vi "NI9239_Producer_Consumer.vi"() -> ()   [LabVIEW 2018]
doc: "Use this template to build a producer/consumer design pattern. Use this template when you need to execute a process, such as data analysis, when a data source, such as a triggered acquisition, produces data at an uneven rate and you need to execute the process when the data becomes available."
uses:
  <vilib>/DAQmx/read.llb/DAQmx Read (Analog 1D Wfm NChan NSamp).vi
  <vilib>/Utility/file.llb/Write Delimited Spreadsheet (string).vi
  <vilib>/DAQmx/miscellaneous.llb/DAQmx Fill In Error Info.vi
  <vilib>/ptbypt/NI_PtbyPt.lvlib
panel:
  out "Directemp (C)":string
  in  "max voltage value":dbl=1.0 format="%0.2f"
  in  "min voltage value":dbl=-1.0 format="%0.2f"
  out "Tot. samples/sec":dbl=1397.9644232175574 format="%_5g"
  out "Array Size":dbl=1000.0
  out "Data Points/Sec":dbl=1.3979644232175574 format="%#_4g"
  in  "samples \nper channel":i32=1000
  in  "samp./ch.":i32=1000
  out "pH output":dbl=3.8843481913333946
  out "error out":errorcluster
  in  "stop":bool
  out "Total Data Points":i32=1166
  out "data":waveform(dbl)[](array[waveform])=[{"t0"=timestamp(3649432382.4522414 s since 1904-01-01), "dt"=0.00062, "Y"=array[1000 elements], "attributes"=variant("NI_ChannelName"=variant(string "Voltage"), "NI_UnitDescription"=variant(string "Volts"))}]
  out "std dev (mV)":dbl=0.018712825305373 format="%0.4f"
  in  "stdev samples":i32=100
  out "Voltage":dbl[][](array[numeric])=[[-0.1627778496], [-0.162776595675], [-0.16276029465], [-0.162771579975], [-0.162937098075], [-0.163070014125], [-0.16318662915], [-0.163360924725], [-0.16341985920000002], [-0.163636788225], [-0.163847447625], [-0.16384870155], [-0.1640969787], [-0.164038044225], [-0.164186007375], [-0.16422487905], [-0.16418475345], [-0.164040552075], [-0.163872526125], [-0.16373459437500001], [-0.163659358875], [-0.16361797935], [-0.163498856475], [-0.16323177045], [-0.162989762925], [-0.162989762925], [-0.1628932107], [-0.16271515335], [-0.162728946525], [-0.1627728339], [-0.162756532875], [-0.1629533991], [-0.16315402710000002], [-0.1632443097], [-0.163333338375], [-0.16343741415000002], [-0.16373584830000001], [-0.163947761625], [-0.16401421965000001], [-0.1641170415], [-0.1641972927], [-0.16433522445], [-0.164223625125], [-0.1641521514], [-0.164103248325], [-0.16398914115000002], [-0.1638261309], [-0.16371076980000002], [-0.16358286945], [-0.163365940425], [-0.1630988544], [-0.163012333575], [-0.16287816360000001], [-0.16283051445], [-0.162787881], [-0.162787881], [-0.162723930825], [-0.16286186257500002], [-0.163002302175], [-0.1631139015], [-0.163197914475], [-0.16327691175], [-0.16339728855], [-0.163691960925], [-0.163852463325], [-0.163980363675], [-0.164110771875], [-0.164108264025], [-0.16428757530000002], [-0.16424494185], [-0.164168452425], [-0.16408945515], [-0.163952777325], [-0.16377848175], [-0.1636555971], [-0.163461238725], [-0.163373463975], [-0.1631740899], [-0.16308631515], [-0.162934590225], [-0.16287690967500001], [-0.162746501475], [-0.162676281675], [-0.162733962225], [-0.162756532875], [-0.1630186032], [-0.16309133085], [-0.16329697455], [-0.1633596708], [-0.1635101418], [-0.16373208652500001], [-0.163910143875], [-0.164075661975], [-0.16415465925], [-0.164173468125], [-0.164183499525], [-0.1642073241], [-0.16412958075], [-0.1639665705], [-0.16393396845], [-0.163807322025], [-0.163679421675], [-0.16342863667500002], [-0.163303244175], [-0.163042427775], [-0.16295590695], [-0.16280042025], [-0.162759040725], [-0.16267502775], [-0.1626273786], [-0.1626574728], [-0.162696344475], [-0.16284806940000002], [-0.163052459175], [-0.16321170765], [-0.1633697022], [-0.163413589575], [-0.1637709582], [-0.16382863875], [-0.1639465077], [-0.164085693375], [-0.16418475345], [-0.16419478485], [-0.16426500465], [-0.16426500465], [-0.164043059925], [-0.163867510425], [-0.1638461937], [-0.1636606128], [-0.163488825075], [-0.163288197075], [-0.16306123665], [-0.162999794325], [-0.16285433902500002], [-0.162919543125], [-0.162708883725], [-0.16272518475], [-0.16279540455], [-0.1628029281], [-0.162982239375], [-0.1631991684], [-0.16329195885], [-0.163330830525], [-0.16356280665], [-0.163774719975], [-0.16384870155], [-0.16400544217500002], [-0.164063122725], [-0.1641722142], [-0.164193530925], [-0.16419980055], [-0.164133342525], [-0.164043059925], [-0.163932714525], [-0.163696976625], [-0.16364807355], [-0.163543997775], [-0.163189137], [-0.163115155425], [-0.162942113775], [-0.1629032421], [-0.162781611375], [-0.162686313075], [-0.16277032605], [-0.16265496495], [-0.162821736975], [-0.162969700125], [-0.163127694675], [-0.16315653495000002], [-0.163406066025], [-0.1635703302], [-0.16384368585], [-0.16389885855], [-0.16404431385], [-0.164073154125], [-0.164211085875], [-0.1642023084], [-0.164213593725], [-0.164251211475], [-0.16410951795], [-0.163875033975], [-0.163777227825], [-0.16367816775], [-0.16344493770000001], [-0.16315402710000002], [-0.1630687602], [-0.162984747225], [-0.16286687827500002], [-0.16281546735], [-0.1626023001], [-0.162789134925], [-0.16276531035], [-0.16293584415], [-0.163077537675], [-0.16316656635000001], [-0.163230516525], [-0.1633245609], [-0.163676913825], [-0.163802306325], [-0.163950269475], [-0.164113279725], [-0.1640769159], [-0.164253719325], [-0.16428632137500002], [-0.16429384492500002], [-0.1641521514], [-0.1640568531], [-0.163865002575], [-0.16376343465], [-0.1636756599], [-0.1635753459], [-0.16320167625], [-0.163044935625], [-0.1628982264], [-0.162838038], [-0.162751517175], [-0.1626825513], [-0.162708883725], [-0.162668758125], [-0.16292581275], [-0.163019857125], [-0.16316782027500001], [-0.163300736325], [-0.163388511075], [-0.1637759739], [-0.16393396845], [-0.16401547357500001], [-0.1640618688], [-0.1641070101], [-0.164206070175], [-0.16423491045], [-0.16422989475], [-0.164191023075], [-0.16402048927500001], [-0.1638863193], [-0.163782243525], [-0.16364807355], [-0.16342612882500002], [-0.163075029825], [-0.163049951325], [-0.16294085985], [-0.162829260525], [-0.1628280066], [-0.16277534175], [-0.16276531035], [-0.162809197725], [-0.1628330223], [-0.16303615815], [-0.16312142505], [-0.16330700595], [-0.1633847493], [-0.163596662625], [-0.16390387425], [-0.1639314606], [-0.1641019944], [-0.16407440805], [-0.1641772299], [-0.16413961215], [-0.164266258575], [-0.164118295425], [-0.16395403125], [-0.163774719975], [-0.163679421675], [-0.163579107675], [-0.1634148435], [-0.16313396430000002], [-0.16301609535], [-0.16285183117500002], [-0.16295590695], [-0.162794150625], [-0.162721422975], [-0.162806689875], [-0.162826752675], [-0.162977223675], [-0.16302111105], [-0.16316029672500001], [-0.1632142155], [-0.16344869947500001], [-0.16379352885], [-0.1639866333], [-0.164080677675], [-0.1641170415], [-0.16419980055], [-0.164246195775], [-0.16425998895], [-0.164233656525], [-0.164143373925], [-0.1639264449], [-0.1638110838], [-0.16365308925], [-0.163584123375], [-0.163386003225], [-0.163070014125], [-0.1630286346], [-0.1628129595], [-0.16285057725000002], [-0.162784119225], [-0.1627527711], [-0.1627026141], [-0.162814213425], [-0.1629333363], [-0.16314274177500002], [-0.16323678615], [-0.163345877625], [-0.163541489925], [-0.16384870155], [-0.16388882715], [-0.164093216925], [-0.164188515225], [-0.164241180075], [-0.164261242875], [-0.164198546625], [-0.164138358225], [-0.164110771875], [-0.1639063821], [-0.1638512094], [-0.16373710222500001], [-0.16366312065], [-0.16335716295], [-0.163077537675], [-0.1629935247], [-0.16287189397500001], [-0.1627678182], [-0.16268004345], [-0.162696344475], [-0.162718915125], [-0.16283553015], [-0.16290073425], [-0.163175343825], [-0.163230516525], [-0.163323306975], [-0.1635151575], [-0.1638110838], [-0.1639063821], [-0.1641220572], [-0.164065630575], [-0.16415967495], [-0.164258735025], [-0.16419478485], [-0.1641822456], [-0.1641019944], [-0.163891335], [-0.163819861275], [-0.163621741125], [-0.163596662625], [-0.163401050325], [-0.1630988544], [-0.1629985404], [-0.162771579975], [-0.16277534175], [-0.16267502775], [-0.1628430537], [-0.16272518475], [-0.162838038], [-0.162982239375], [-0.16315778887500001], [-0.163212961575], [-0.163263118575], [-0.163538982075], [-0.16380356025], [-0.163912651725], [-0.1641120258], [-0.16413459645], [-0.16430763810000001], [-0.1644129678], [-0.164173468125], [-0.1642173555], [-0.163972840125], [-0.163891335], [-0.163792274925], [-0.163636788225], [-0.163554029175], [-0.163238040075], [-0.1631239329], [-0.1630035561], [-0.16280042025], [-0.162838038], [-0.162671265975], [-0.16280042025], [-0.16273020045], [-0.162804182025], [-0.162938352], [-0.16315402710000002], [-0.163278165675], [-0.16334211585], [-0.163554029175], [-0.1638010524], [-0.163907636025], [-0.164033028525], [-0.16401421965000001], [-0.16412958075], [-0.16416970635], [-0.164138358225], [-0.164175975975], [-0.16401171180000002], [-0.1639013664], [-0.163649327475], [-0.163518919275], [-0.16349760255], [-0.16316531242500001], [-0.162937098075], [-0.162937098075], [-0.16285559295000002], [-0.16281546735], [-0.162687567], [-0.162681297375], [-0.16270010625], [-0.162819229125], [-0.162932082375], [-0.163057474875], [-0.16313898000000002], [-0.1632593568], [-0.163488825075], [-0.163832400525], [-0.16397409405], [-0.16400042647500002], [-0.1640317746], [-0.16421484765], [-0.1642023084], [-0.1642675125], [-0.164248703625], [-0.16399666470000002], [-0.1638612408], [-0.16372456297500002], [-0.1635803616], [-0.16348757115], [-0.16321170765], [-0.1630838073], [-0.162909511725], [-0.1627928967], [-0.162781611375], [-0.162723930825], [-0.162733962225], [-0.1627226769], [-0.162829260525], [-0.16303114245], [-0.163115155425], [-0.1632693882], [-0.1633646865], [-0.1635552831], [-0.1639565391], [-0.163912651725], [-0.16414964355], [-0.164160928875], [-0.1642574811], [-0.1641571671], [-0.1642073241], [-0.164183499525], [-0.16392895275], [-0.16385371725], [-0.163777227825], [-0.163629264675], [-0.163481301525], [-0.163087569075], [-0.1630286346], [-0.1629533991], [-0.1629935247], [-0.1628179752], [-0.162733962225], [-0.162787881], [-0.162794150625], [-0.16284932332500002], [-0.163072521975], [-0.16314399570000002], [-0.163353401175], [-0.1633646865], [-0.16371578550000002], [-0.163865002575], [-0.16401798142500001], [-0.1640468217], [-0.16402926675], [-0.164242434], [-0.16422487905], [-0.1641270729], [-0.164113279725], [-0.1640317746], [-0.163890081075], [-0.1637609268], [-0.1635954087], [-0.163491332925], [-0.16316029672500001], [-0.1629584148], [-0.162891956775], [-0.162919543125], [-0.162759040725], [-0.1626574728], [-0.162701360175], [-0.162743993625], [-0.162816721275], [-0.163072521975], [-0.1631139015], [-0.16327691175], [-0.16333710015], [-0.16373835615000001], [-0.16390387425], [-0.1639314606], [-0.16404932955], [-0.16417973775], [-0.1642675125], [-0.164218609425], [-0.16423992615], [-0.164196038775], [-0.163902620325], [-0.163887573225], [-0.16373584830000001], [-0.16348757115], [-0.163355909025], [-0.16305120525], [-0.163027380675], [-0.162886941075], [-0.162806689875], [-0.1627678182], [-0.1626975984], [-0.16275527895], [-0.16273521615], [-0.162967192275], [-0.163029888525], [-0.163170328125], [-0.1632994824], [-0.163523934975], [-0.163769704275], [-0.163985379375], [-0.164090709075], [-0.164120803275], [-0.164041806], [-0.164221117275], [-0.1641521514], [-0.164206070175], [-0.164105756175], [-0.16386374865], [-0.163817353425], [-0.16362801075], [-0.16352769675], [-0.16338224145], [-0.163087569075], [-0.163088823], [-0.16294085985], [-0.16286687827500002], [-0.16276029465], [-0.162741485775], [-0.16273020045], [-0.16273521615], [-0.1628982264], [-0.163070014125], [-0.1632041841], [-0.163310767725], [-0.1635101418], [-0.1637809896], [-0.163917667425], [-0.163970332275], [-0.164108264025], [-0.1640819316], [-0.16424995755], [-0.164168452425], [-0.16428506745000002], [-0.164183499525], [-0.16400795002500002], [-0.163857479025], [-0.163794782775], [-0.16355277525], [-0.16331703735], [-0.162984747225], [-0.163115155425], [-0.162787881], [-0.16281045165], [-0.16266499635], [-0.162749009325], [-0.162819229125], [-0.162766564275], [-0.1629032421], [-0.1631841213], [-0.16332706875], [-0.1633596708], [-0.16352769675], [-0.163847447625], [-0.163837416225], [-0.16388381145], [-0.16400669610000002], [-0.164196038775], [-0.16430889202500001], [-0.16423491045], [-0.16423491045], [-0.16401923535000001], [-0.16390387425], [-0.163779735675], [-0.163654343175], [-0.163556537025], [-0.163310767725], [-0.163115155425], [-0.16295590695], [-0.16290574995], [-0.1628229909], [-0.162676281675], [-0.1626624885], [-0.16262988645], [-0.162718915125], [-0.16293584415], [-0.163034904225], [-0.163212961575], [-0.16342236705000002], [-0.16347753975], [-0.1638863193], [-0.163975347975], [-0.164030520675], [-0.1641070101], [-0.16419478485], [-0.16428005175000002], [-0.16424494185], [-0.16427879782500002], [-0.164095724775], [-0.1639314606], [-0.16379352885], [-0.16367315205], [-0.163518919275], [-0.163245563625], [-0.162947129475], [-0.162994778625], [-0.16286687827500002], [-0.16287565575000001], [-0.16270512195], [-0.1626775356], [-0.162736470075], [-0.162756532875], [-0.1629935247], [-0.163087569075], [-0.163192898775], [-0.163383495375], [-0.16355779095], [-0.163915159575], [-0.163900112475], [-0.164145881775], [-0.164113279725], [-0.164163436725], [-0.164231148675], [-0.164180991675], [-0.164075661975], [-0.163920175275], [-0.163844939775], [-0.163740864], [-0.16364807355], [-0.1635151575], [-0.163212961575], [-0.163097600475], [-0.16302612675], [-0.162884433225], [-0.16285057725000002], [-0.16276531035], [-0.162791642775], [-0.162703868025], [-0.16287565575000001], [-0.163070014125], [-0.163185375225], [-0.1632142155], [-0.163353401175], [-0.163590393], [-0.163789767075], [-0.163970332275], [-0.1640568531], [-0.1640618688], [-0.164251211475], [-0.16428130567500002], [-0.16417472205], [-0.164168452425], [-0.16393396845], [-0.163852463325], [-0.163764688575], [-0.16360794795], [-0.163496348625], [-0.163195406625], [-0.16309133085], [-0.162957160875], [-0.162934590225], [-0.162683805225], [-0.1628079438], [-0.162687567], [-0.162741485775], [-0.16285559295000002], [-0.162999794325], [-0.163105124025], [-0.1632192312], [-0.163350893325], [-0.1635151575], [-0.163812337725], [-0.163841178], [-0.16414964355], [-0.1640719002], [-0.1641972927], [-0.1642474497], [-0.164241180075], [-0.16414964355], [-0.1640518374], [-0.1638813036], [-0.16388381145], [-0.163644311775], [-0.1635101418], [-0.163122678975], [-0.163064998425], [-0.1629283206], [-0.162824244825], [-0.162789134925], [-0.16264493355], [-0.162761548575], [-0.16273521615], [-0.162909511725], [-0.1630186032], [-0.163200422325], [-0.1632643725], [-0.16344493770000001], [-0.16367816775], [-0.16377848175], [-0.16399541077500002], [-0.164060614875], [-0.164108264025], [-0.16418475345], [-0.164213593725], [-0.164238672225], [-0.16411954935], [-0.1639615548], [-0.163872526125], [-0.163689453075], [-0.1635302046], [-0.16331703735], [-0.16312644075], [-0.16306625235], [-0.16290574995], [-0.16285684687500002], [-0.162804182025], [-0.162687567], [-0.16269007485], [-0.162751517175], [-0.1629584148], [-0.16315402710000002], [-0.16316782027500001], [-0.163278165675], [-0.163383495375], [-0.163621741125], [-0.1638361623], [-0.163960300875], [-0.16401045787500002], [-0.164060614875], [-0.16427879782500002], [-0.164120803275], [-0.1641872613], [-0.164085693375], [-0.163875033975], [-0.16382863875], [-0.16372581690000002], [-0.16357283805], [-0.16343365237500002], [-0.16315151925000002], [-0.16300104825], [-0.16294085985], [-0.16281546735], [-0.1627126455], [-0.1626775356], [-0.16266499635], [-0.16276531035], [-0.1628029281], [-0.1630637445], [-0.1632593568], [-0.163333338375], [-0.1634599848], [-0.163659358875], [-0.1638662565], [-0.163915159575], [-0.164068138425], [-0.164085693375], [-0.164313907725], [-0.164208578025], [-0.164211085875], [-0.164133342525], [-0.163885065375], [-0.1638612408], [-0.1636957227], [-0.1635001104], [-0.163391018925], [-0.1630737759], [-0.1630687602], [-0.1629584148], [-0.16291076565], [-0.162743993625], [-0.1627527711], [-0.162738977925], [-0.1627226769], [-0.163004810025], [-0.163105124025], [-0.163197914475], [-0.16331703735], [-0.163488825075], [-0.163804814175], [-0.163892588925], [-0.16400669610000002], [-0.16414462785], [-0.164143373925], [-0.1643678265], [-0.16418976915], [-0.1642324026], [-0.16402926675], [-0.163910143875], [-0.163817353425], [-0.16365308925], [-0.163611709725], [-0.163289451], [-0.163088823], [-0.16308129945], [-0.16288192537500001], [-0.162794150625], [-0.162713899425], [-0.162728946525], [-0.162731454375], [-0.162769072125], [-0.162949637325], [-0.16307628375], [-0.163182867375], [-0.16339728855], [-0.16342863667500002], [-0.16372957867500001], [-0.163907636025], [-0.1640719002], [-0.164103248325], [-0.164168452425], [-0.164236164375], [-0.1641320886], [-0.1642223712], [-0.164050583475], [-0.163852463325], [-0.163817353425], [-0.163596662625], [-0.163468762275], [-0.1632342783], [-0.162967192275], [-0.163110139725], [-0.16286060865000002], [-0.16285684687500002], [-0.162698852325], [-0.16271013765], [-0.16273020045], [-0.162761548575], [-0.163024872825], [-0.16313521822500002], [-0.163250579325], [-0.163348385475], [-0.1635251889], [-0.1638060681], [-0.163867510425], [-0.16397910975], [-0.1640769159], [-0.164238672225], [-0.16428005175000002], [-0.1641671985], [-0.164238672225], [-0.16406437665], [-0.163847447625], [-0.163774719975], [-0.1635853773], [-0.16350261825], [-0.163260610725], [-0.1630737759], [-0.1630186032], [-0.16287941752500001], [-0.162909511725], [-0.162749009325], [-0.162751517175], [-0.1627728339], [-0.16289070285], [-0.163014841425], [-0.16306123665], [-0.16325684895], [-0.1633847493], [-0.16357785375], [-0.1638010524], [-0.163917667425], [-0.164033028525], [-0.164068138425], [-0.164143373925], [-0.1641722142], [-0.16421484765], [-0.1641822456], [-0.1639264449], [-0.1638863193], [-0.163740864], [-0.163533966375], [-0.16352268105], [-0.1632543411], [-0.16304117385], [-0.16292079705], [-0.162781611375], [-0.162799166325], [-0.162751517175], [-0.162799166325], [-0.162703868025], [-0.162841799775], [-0.163004810025], [-0.163182867375], [-0.163222992975], [-0.1633697022], [-0.163616725425], [-0.16384870155], [-0.163897604625], [-0.1641170415], [-0.1641170415], [-0.1641671985], [-0.164231148675], [-0.1641471357], [-0.16412958075], [-0.1639665705], [-0.16388381145], [-0.163804814175], [-0.1635201732], [-0.163523934975], [-0.1631289486], [-0.1630737759], [-0.162899480325], [-0.162904496025], [-0.162787881], [-0.16273020045], [-0.16279038885], [-0.1628029281], [-0.16297095405], [-0.163057474875], [-0.16315026532500002], [-0.1632844353], [-0.16333710015], [-0.163551521325], [-0.163872526125], [-0.16383867015], [-0.164206070175], [-0.1642223712], [-0.164243687925], [-0.164241180075], [-0.1642725282], [-0.16423491045], [-0.1640267589], [-0.163935222375], [-0.16376343465], [-0.163691960925], [-0.163408573875], [-0.16307126805], [-0.16301107965], [-0.162947129475], [-0.162814213425], [-0.1627176612], [-0.16273020045], [-0.16269007485], [-0.16263741], [-0.16280042025], [-0.163054967025], [-0.16319666055], [-0.163260610725], [-0.16334211585], [-0.16376343465], [-0.16400168040000002], [-0.16395403125], [-0.16410951795], [-0.1641872613], [-0.164168452425], [-0.164216101575], [-0.1641822456], [-0.16409447085], [-0.16394399985], [-0.1638963507], [-0.16375841895], [-0.16360794795], [-0.1634700162], [-0.16320669195], [-0.163052459175], [-0.1628932107], [-0.16287816360000001], [-0.1626975984], [-0.162686313075], [-0.162733962225], [-0.1627276926], [-0.162909511725], [-0.163062490575], [-0.163059982725], [-0.16329195885], [-0.163343369775], [-0.1636255029], [-0.163870018275], [-0.163960300875], [-0.16411453365], [-0.164180991675], [-0.16430513025000001], [-0.164198546625], [-0.164150897475], [-0.164033028525], [-0.163977855825], [-0.163804814175], [-0.1636606128], [-0.1636004244], [-0.16338224145], [-0.163072521975], [-0.163004810025], [-0.162901988175], [-0.162774087825], [-0.16265998065], [-0.162726438675], [-0.16267502775], [-0.162708883725], [-0.1627728339]]
  out "Chart":dbl(graph)=-0.1634697603993
  out "Time":string="12:13:03 "
  out "Date":string="23/08/19 "
  in  "Write to SS?":bool
  in  "Data Save":path=path "C:/Users/pjbre/Documents/Labview VI's/NI 9239 Data Logger/Durafet_Voltages.csv"
  in  "rate (Hz)":dbl=10.0
  # "Producer"
  # "Consumer"
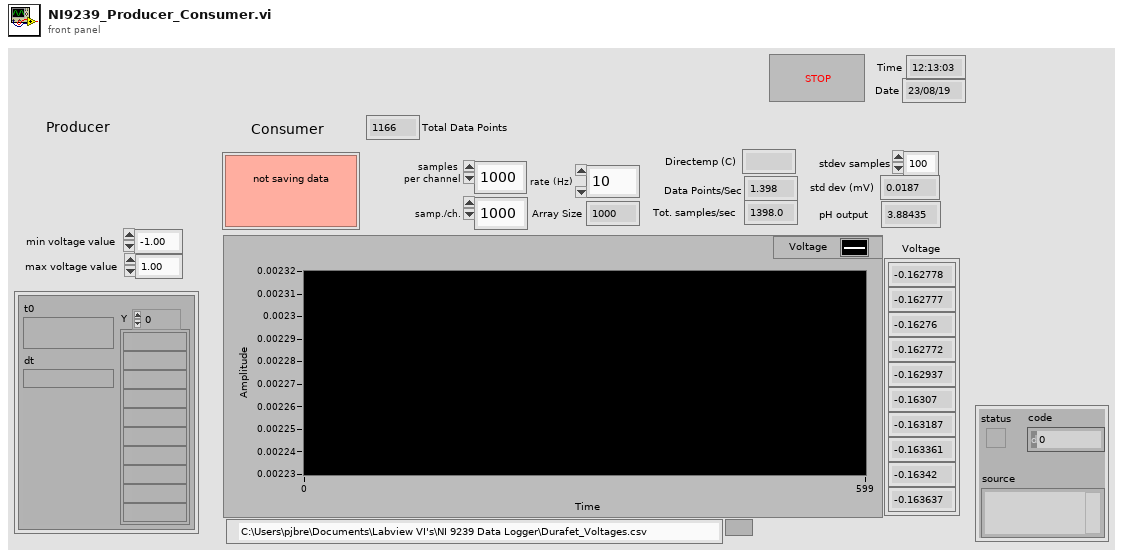
[diagram p1: front panel]
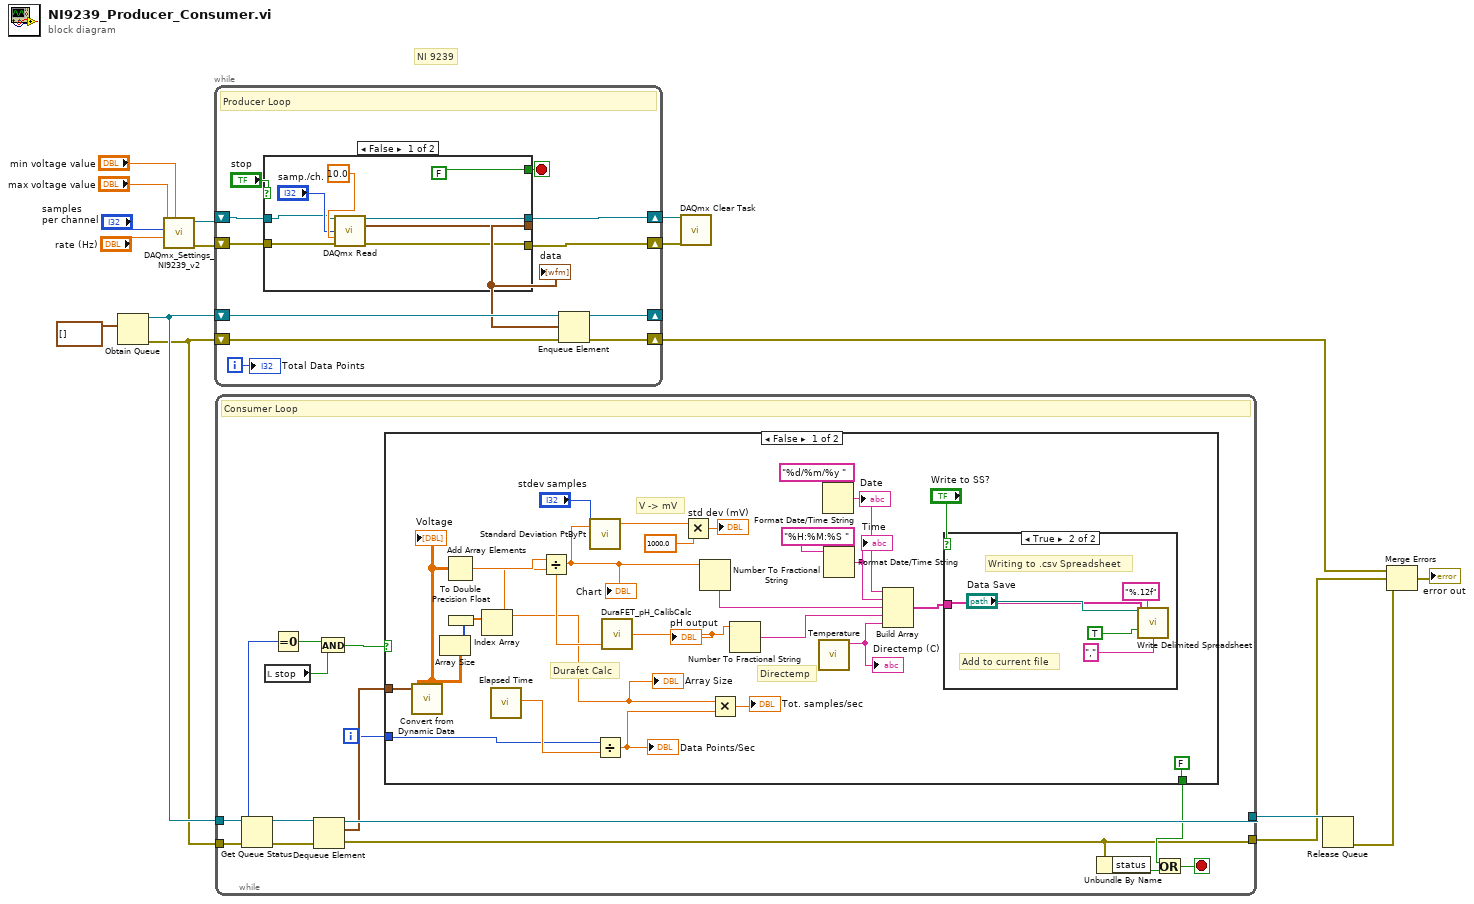
[diagram p0: block diagram]
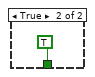
[diagram p3: hidden frame]
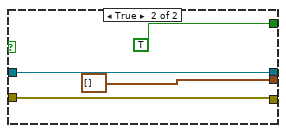
[diagram p4: hidden frame]
diagram:
  # "NI 9239"
  n1 = Obtain Queue(element data type=waveform(dbl)[] [] ("data")) -> (queue out=w16:refnum<queue>, error out=w12:errorcluster)  [unwired: 3 in, 2 out]
  n2 = call "DAQmx_Settings_NI9239_v2.vi"("minimum value"="min voltage value", "rate"="rate (Hz)", "samples per channel"="samples \nper channel", "maximum value"="max voltage value") -> ("error out"=w5:errorcluster, "task out"=w6:refnum<k21>)  [unwired: 6 in]
  n3 = while {
    shift-right: [w25] -> w9
    shift-left: w12 -> [w26]
    shift-right: [w27] -> _
    shift-left: w16 -> [w28]
    shift-right: [w22] -> w8
    shift-left: w6 -> [w24]
    shift-right: [w21] -> w7
    shift-left: w5 -> [w23]
    i -> [w19]
    stop <- w17 stop-if-true
    # "Producer Loop"
    n4 = case shown="False" "stop" {
      tunnel: w24 -> [w29 w39]
      tunnel: w23 -> [w32 w38]
      tunnel: [w35 w39] -> w22
      tunnel: [w33 w38] -> w21
      tunnel: [w34 waveform(dbl)[] [] ("data")] -> w20
      tunnel: [FALSE TRUE] -> w17
      frame False {
        n5 = call-poly <vilib>:"DAQmx Read.vi"("task/channels in"=w29, "number of samples per channel"="samp./ch.", "timeout"=10.0 ("timeout (s)"), "error in"=w32) -> ("task out"=w35:refnum<k21>, "data"=w34:waveform(dbl)[], "error out"=w33:errorcluster)  [unwired: 9 in]
      }
      frame True {
      }
    }
    "data" <- w20
    n6 = Enqueue Element(queue=w28, element=w20, error in (no error)=w26) -> (queue out=w27:refnum<queue>, error out=w25:errorcluster)  [unwired: 2 out]
    "Total Data Points" <- w19
  }
  n7 = while {
    tunnel: w16 -> [w47]
    tunnel: [w54] -> w11
    tunnel: w12 -> [w50]
    tunnel: [w49] -> w10
    i -> [w41]
    stop <- w52 stop-if-true
    # "Consumer Loop"
    n8 = Get Queue Status(queue=w47) -> (queue out=w46:refnum<queue>, # elements in queue=w44:i32)  [unwired: 2 in, 6 out]
    n9 = local read "stop"() -> (w42:bool)
    n10 = Equal To 0?(x=w44) -> (x = 0?=w45:bool)
    n11 = Dequeue Element(queue=w46, error in (no error)=w50) -> (queue out=w54:refnum<queue>, element=w48:waveform(dbl)[], error out=w49:errorcluster)  [unwired: 2 out]
    n12 = And(x=w45, y=w42) -> (x .and. y?=w43:bool)
    n13 = case shown="False" w43 {
      tunnel: [FALSE TRUE] -> w51
      tunnel: w48 -> [w61 _]
      tunnel: w41 -> [w57 _]
      frame False {
        # "Directemp"
        # "V -> mV"
        # "Durafet Calc"
        n14 = call "Convert from Dynamic Data"("Dynamic Data Type"=w61) -> ("Array"=w63:dbl[][])  [unwired: 3 in]
        "Voltage" <- w63
        n15 = Array Size(array=w63) -> (size(s)=w65:i32[])
        n16 = Add Array Elements(numeric array=w63) -> (sum=w74:dbl)
        n17 = To Double Precision Float(number=w65) -> (double precision float=w64:dbl[])
        n18 = Index Array(array=w64) -> (element=w56:dbl)  [unwired: 1 in]
        "Array Size" <- w56
        n19 = call "Elapsed Time"() -> ("Elapsed Time (s)"=w60:dbl)  [unwired: 12 in, 7 out]
        n20 = Divide(x=w74, y=w56) -> (x/y=w70:dbl)
        "Chart" <- w70
        n21 = call <vilib>:"Standard Deviation PtByPt.vi"("x"=w70, "sample length"="stdev samples") -> ("standard deviation"=w66:dbl)  [unwired: 1 in, 2 out]
        n22 = Divide(x=w57, y=w60) -> (x/y=w59:dbl)
        "Data Points/Sec" <- w59
        n23 = call "DuraFET_pH_CalibCalc.vi"("Eint: (mean voltage)"=w70) -> ("pHint_tot"=w71:dbl)  [unwired: 2 in]
        "pH output" <- w71
        n24 = Multiply(x=w66, y=1000.0) -> (x*y=→"std dev (mV)":dbl)
        n25 = Number To Fractional String(number=w70) -> (F-format string=w73:string)  [unwired: 3 in]
        n26 = Multiply(x=w56, y=w59) -> (x*y=→"Tot. samples/sec":dbl)
        n27 = Number To Fractional String(number=w71) -> (F-format string=w72:string)  [unwired: 3 in]
        n28 = call "Temperature.vi"() -> ("read buffer"=w55:string)  [unwired: 11 in]
        "Directemp (C)" <- w55
        n29 = Format Date/Time String(time format string (%c)="%d/%m/%y ") -> (date/time string=w78:string)  [unwired: 2 in]
        "Date" <- w78
        n30 = Format Date/Time String(time format string (%c)="%H:%M:%S ") -> (date/time string=w77:string)  [unwired: 2 in]
        "Time" <- w77
        n31 = Build Array(w78, w77, w73, w72, w55) -> (w80:string[])
        n32 = case shown="True" "Write to SS?" {
          tunnel: w80 -> [_ w81]
          frame False {
          }
          frame True {
            # "Add to current file"
            # "Writing to .csv Spreadsheet"
            n33 = call-poly <vilib>:"Write Delimited Spreadsheet.vi"("file path (dialog if empty)"="Data Save", "format (%s)"="%.12f" ("format (%.3f)"), "1D data"=w81, "append to file? (new file:F)"=TRUE, "delimiter (\\t)"="," ("delimiter (\\t)")) -> ()  [unwired: 9 in, 2 out]
          }
        }
      }
      frame True {
      }
    }
    n34 = Unbundle By Name(w49) -> ("status"=w53:bool)
    n35 = Or(x=w51, y=w53) -> (x .or. y?=w52:bool)
  }
  n36 = call <vilib>:"DAQmx Clear Task.vi"("task in"=w8, "error in"=w7) -> ()  [unwired: 13 in, 1 out]
  n37 = Release Queue(queue=w11) -> (error out=w13:errorcluster)  [unwired: 2 in, 2 out]
  n38 = Merge Errors(w9, w10, w13) -> (→"error out":errorcluster)
